vi "Triax320 SetSlits.vi"(6 "Slit":enum16{"Input", "Output", "Both"}(ring), 8 "error in (no error)":errorcluster, 9 "OutSlit":dbl caption="Output Slit (mm)" min=0.0 max=10.0 step=0.001 format="%.3f", 10 "InSlit":dbl caption="Input Slit (mm)" min=0.0 max=10.0 step=0.001 format="%.3f", 11 "Triax VISA Rsrc":refnum<visa-resource-name>="SR530") -> (0 "error out":errorcluster, 1 "OutSlit Out":dbl caption="Output Slit (mm)" min=0.0 max=10.0 step=0.001 format="%.3f", 2 "InSlit Out":dbl caption="Input Slit (mm)" min=0.0 max=10.0 step=0.001 format="%.3f", 3 "Triax VISA Rsrc Out":refnum<visa-resource-name>="SR530")   [LabVIEW 2019]
uses:
  <userlib>/Triax320/TriaxParams.ctl
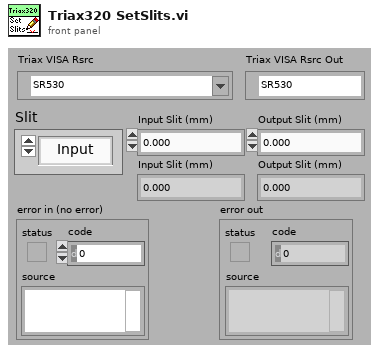
[diagram p1: front panel]
types:
  T1 = typedef "TriaxParams.ctl" = enum16{"Grating", "CalOffset", "Line Density (grv/mm)", "Input Slit (mm)", "Output Slit (mm)", "Both Slit (mm)", "Grating Desc.", "Tous"}
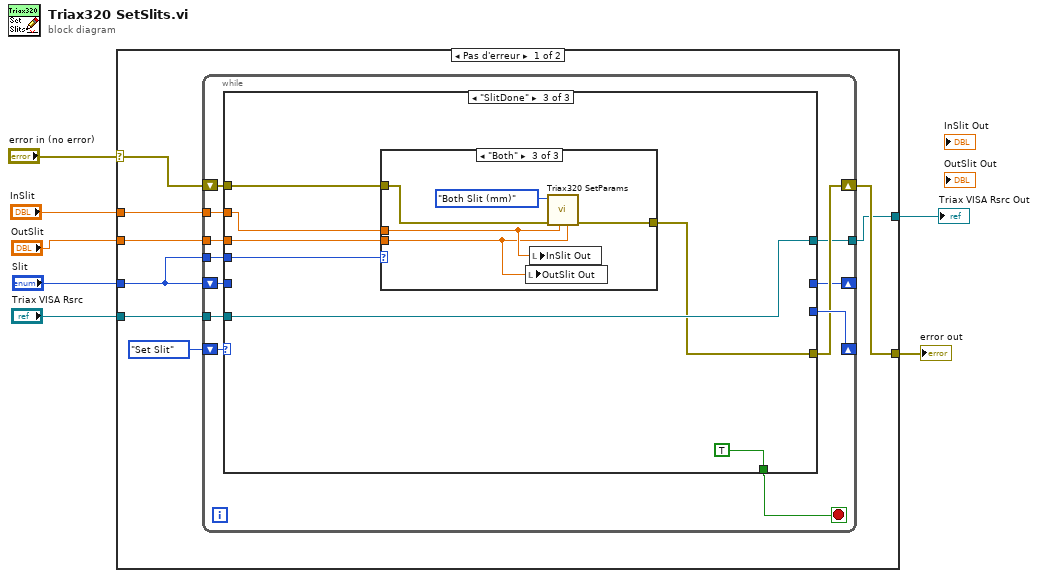
[diagram p0: block diagram]
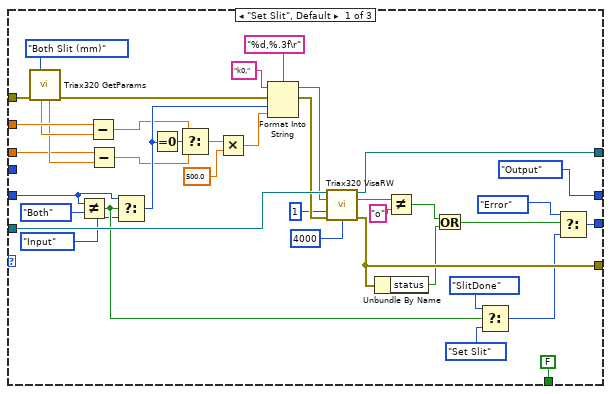
[diagram p2: hidden frame]
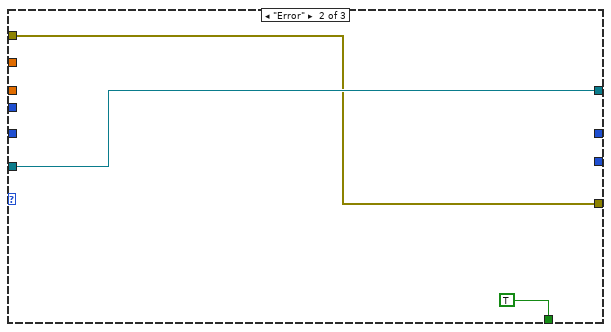
[diagram p3: hidden frame]
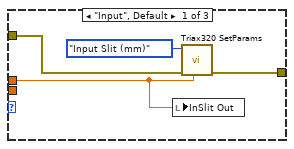
[diagram p4: hidden frame]
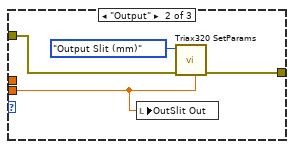
[diagram p5: hidden frame]
diagram:
  n1 = case shown="Pas d'erreur" "error in (no error)" {
    selector: "error in (no error)" -> [w14 w91]
    tunnel: "Triax VISA Rsrc" -> [w15 w90]
    tunnel: [w12 w91] -> w5
    tunnel: [w11 w90] -> w4
    tunnel: "Slit" -> [w8 _]
    tunnel: "InSlit" -> [w10 _]
    tunnel: "OutSlit" -> [w9 _]
    frame No Error {
      n2 = while {
        shift-right: [w25] -> _
        shift-left: enum16{"Error", "Set Slit", "SlitDone"}."Set Slit" -> [w27]
        tunnel: w15 -> [w24]
        shift-right: [w22] -> w12
        shift-left: w14 -> [w23]
        tunnel: [w21] -> w11
        tunnel: w10 -> [w19]
        tunnel: w9 -> [w18]
        shift-right: [w17] -> _
        shift-left: w8 -> [w20]
        tunnel: w8 -> [w16]
        stop <- w26 stop-if-true
        n3 = case shown="\"SlitDone\"" w27 {
          tunnel: [FALSE TRUE TRUE] -> w26
          tunnel: [w64 _ _] -> w25
          tunnel: w24 -> [w66 w69 w76]
          tunnel: w23 -> [w56 w67 w74]
          tunnel: [w43 w67 w73] -> w22
          tunnel: [w65 w69 w76] -> w21
          tunnel: w20 -> [w49 _ _]
          tunnel: w19 -> [w60 _ w70]
          tunnel: w18 -> [w57 _ w71]
          tunnel: [enum16{"Input", "Output", "Both"}."Output" ("Slit") _ _] -> w17
          tunnel: w16 -> [_ _ w72]
          frame "Set Slit", Default {
            n4 = call <userlib>:"Triax320 GetParams.vi"("error in"=w56, "Param"=TriaxParams."Both Slit (mm)") -> ("error out"=w55:errorcluster, "OutSlit"=w58:dbl, "InSlit"=w59:dbl)  [unwired: 4 in, 3 out]
            n5 = Not Equal?(x=w49, y=enum16{"Input", "Output", "Both"}."Both" ("Slit")) -> (x != y?=w36:bool)
            n6 = Subtract(x=w60, y=w59) -> (x-y=w44:dbl)
            n7 = Subtract(x=w57, y=w58) -> (x-y=w45:dbl)
            n8 = Select(t=w49, s=w36, f=enum16{"Input", "Output", "Both"}."Input" ("Slit")) -> (s? t:f=w48:enum16{"Input", "Output", "Both"})
            n9 = Equal To 0?(x=w48) -> (x = 0?=w47:bool)
            n10 = Select(t=w44, s=w47, f=w45) -> (s? t:f=w46:dbl)
            n11 = Multiply(x=w46, y=500.0) -> (x*y=w29:dbl)
            n12 = Format Into String(format string="%d,%.3f\r" ("chaîne"), initial string="k0," ("chaîne"), error in=w55, w48, w29) -> (resulting string=w50:string, error out=w54:errorcluster)
            n13 = call <userlib>:"Triax320 VisaRW.vi"("VISA Rsrc"=w66, "ChaineCom"=w50, "Nbcaract"=u32 1, "error in (no error)"=w54, "Timeout ms"=u32 4000) -> ("VISA Rsrc Out"=w65:refnum<visa-resource-name>, "ChaineRep"=w52:string, "error out"=w43:errorcluster)  [unwired: 5 in, 3 out]
            n14 = Unbundle By Name(w43) -> ("status"=w42:bool)
            n15 = Not Equal?(x=w52, y="o") -> (x != y?=w41:bool)
            n16 = Or(x=w41, y=w42) -> (x .or. y?=w40:bool)
            n17 = Select(t=enum16{"Error", "Set Slit", "SlitDone"}."SlitDone", s=w36, f=enum16{"Error", "Set Slit", "SlitDone"}."Set Slit") -> (s? t:f=w33:enum16{"Error", "Set Slit", "SlitDone"})
            n18 = Select(t=enum16{"Error", "Set Slit", "SlitDone"}."Error", s=w40, f=w33) -> (s? t:f=w64:enum16{"Error", "Set Slit", "SlitDone"})
          }
          frame "Error" {
          }
          frame "SlitDone" {
            n19 = case shown="\"Both\"" w72 {
              tunnel: w74 -> [w79 w84 w89]
              tunnel: [w78 w83 w88] -> w73
              tunnel: w71 -> [_ w81 w85]
              tunnel: w70 -> [w77 _ w86]
              frame "Input", Default {
                n20 = local write "InSlit Out"(w77) -> ()
                n21 = call <userlib>:"Triax320 SetParams.vi"("InSlit"=w77, "error in"=w79, "Param"=TriaxParams."Input Slit (mm)") -> ("error out"=w78:errorcluster)  [unwired: 8 in]
              }
              frame "Output" {
                n22 = local write "OutSlit Out"(w81) -> ()
                n23 = call <userlib>:"Triax320 SetParams.vi"("OutSlit"=w81, "error in"=w84, "Param"=TriaxParams."Output Slit (mm)") -> ("error out"=w83:errorcluster)  [unwired: 8 in]
              }
              frame "Both" {
                n24 = local write "OutSlit Out"(w85) -> ()
                n25 = local write "InSlit Out"(w86) -> ()
                n26 = call <userlib>:"Triax320 SetParams.vi"("OutSlit"=w85, "InSlit"=w86, "error in"=w89, "Param"=TriaxParams."Both Slit (mm)") -> ("error out"=w88:errorcluster)  [unwired: 7 in]
              }
            }
          }
        }
      }
    }
    frame Error {
    }
  }
  "error out" <- w5
  "Triax VISA Rsrc Out" <- w4
